vi "Function.vi"(8 "error in (no error)":errorcluster, 9 "Numeric B":dbl, 10 "Numeric A":timestamp, 11 "Two Terminal in":refnum<class "Add_Time.lvclass">) -> (0 "error out":errorcluster, 2 "Result":timestamp, 3 "Two Terminal out":refnum<class "Add_Time.lvclass">)   [LabVIEW 2021, in "Add_Time.lvclass"]
uses:
  Add_Time.lvclass
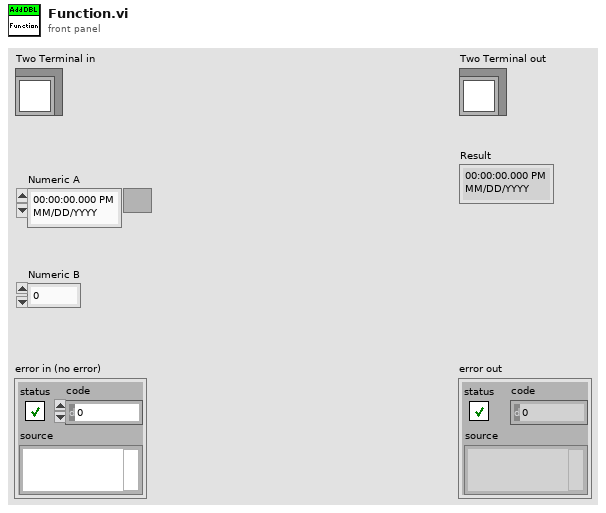
[diagram p1: front panel]
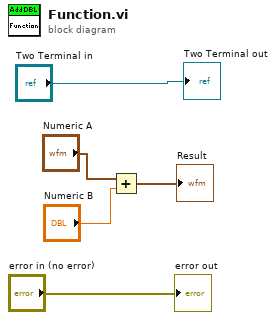
[diagram p0: block diagram]
diagram:
  n1 = Add(x="Numeric A", y="Numeric B") -> (x+y=→"Result":timestamp)
  "error out" <- "error in (no error)"
  "Two Terminal out" <- "Two Terminal in"
